vi "8HP_Clone.vi"(0 "Single 8HP":T1) -> (2 "DAQ Error":errorcluster, 3 "All samples out":sgl[][](array[numeric]), 4 "Ch No":i16[](array[numeric]), 5 "Index":i32[](array[numeric]), 6 "Sampling Rate Hz":dbl)   [LabVIEW 2018]
doc: "Use this plug-in with the Nathan 7609 data acquisition system"
uses:
  Device ID port info.ctl
  ctls/8HP_Cmd (USB).ctl
  Globals/Meas_global.vi
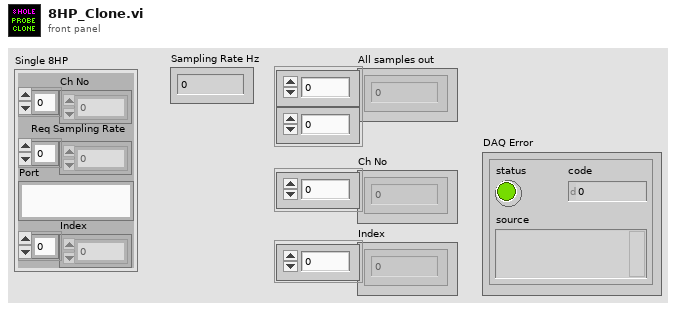
[diagram p1: front panel]
types:
  T1 = typedef "Device ID port info.ctl" = cluster{"Ch No":i16[], "Req Sampling Rate":dbl[], "Port":string, "Index":i32[]}
  T2 = typedef "8HP_Cmd (USB).ctl" = string
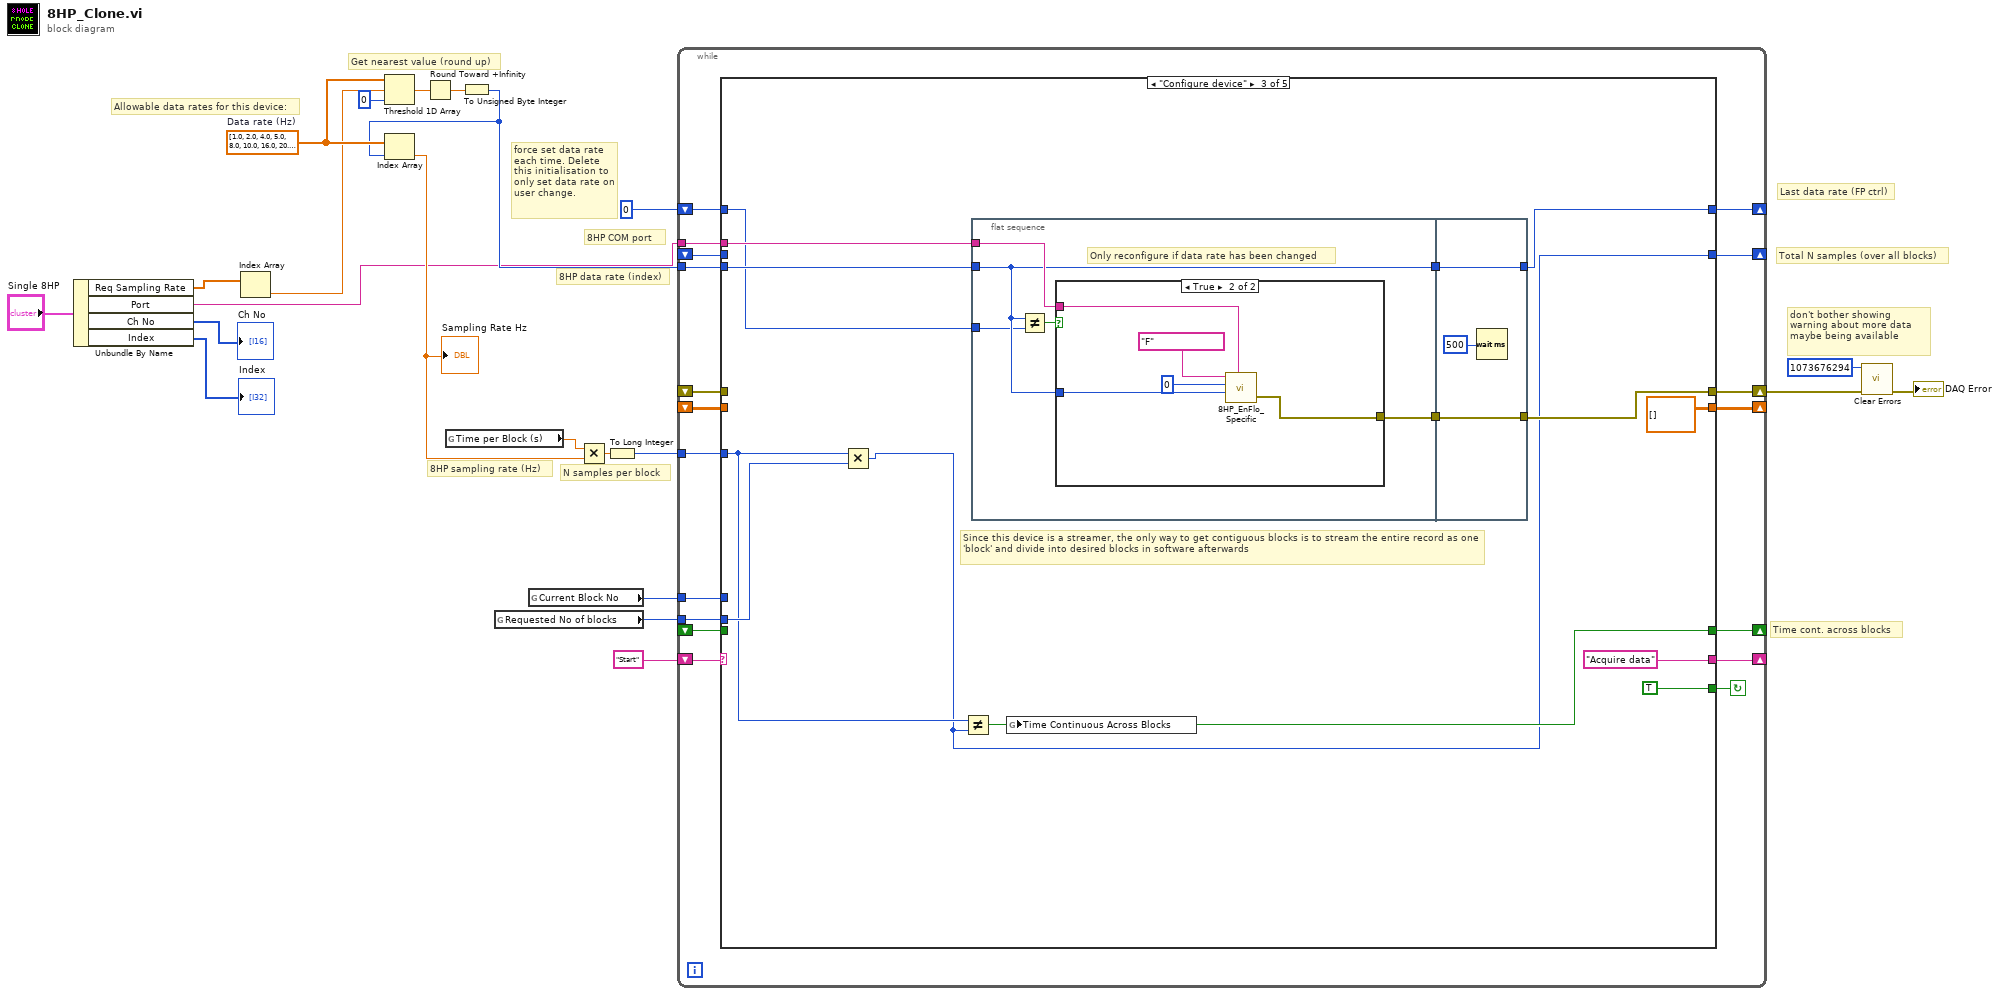
[diagram p0: block diagram]
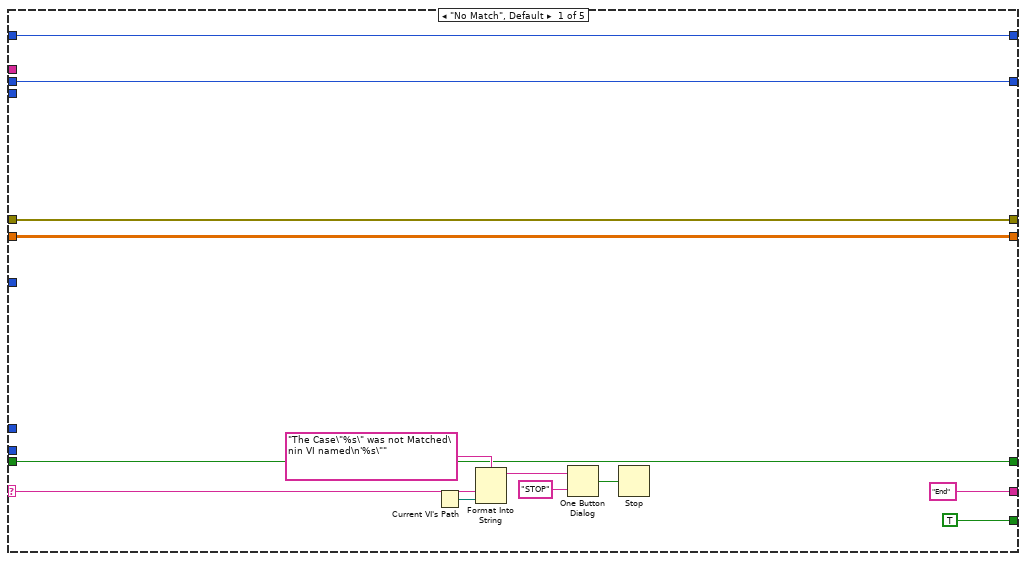
[diagram p2: hidden frame]
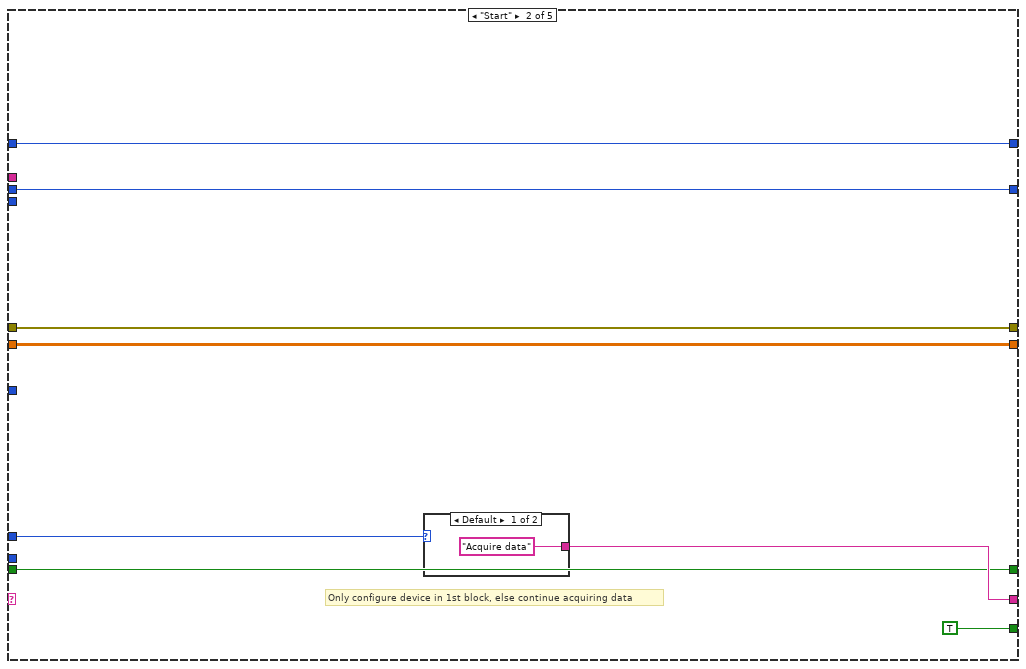
[diagram p3: hidden frame]
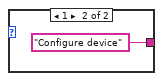
[diagram p4: hidden frame]
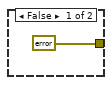
[diagram p5: hidden frame]
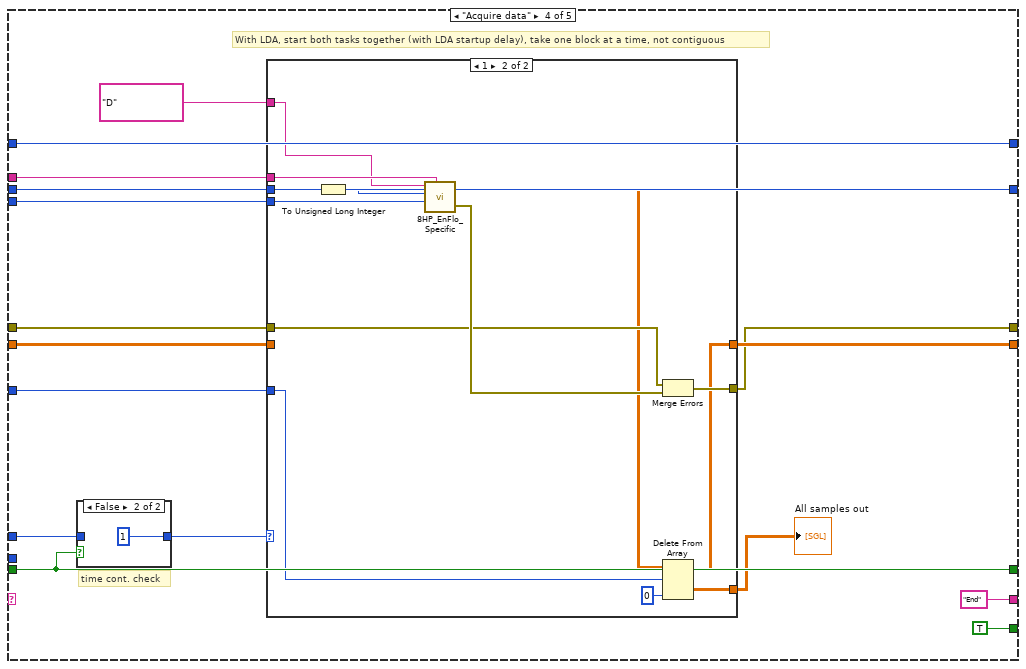
[diagram p6: hidden frame]
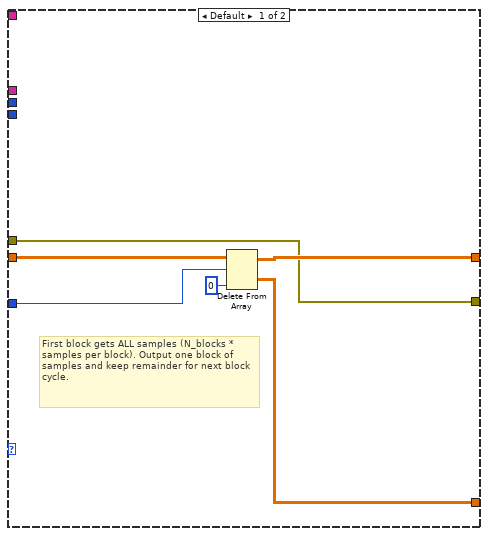
[diagram p8: hidden frame]
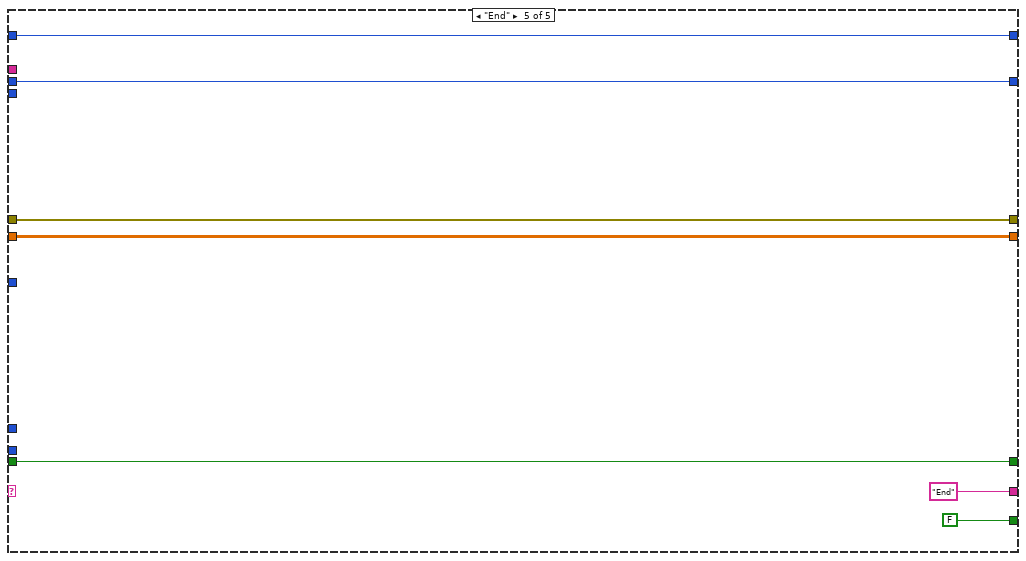
[diagram p9: hidden frame]
diagram:
  w13 = dbl[] [1.0, 2.0, 4.0, 5.0, 8.0, 10.0, 16.0, 20.0, 25.0, 32.0, 40.0, 50.0, 64.0, 80.0, 100.0, 125.0, 160.0, 200.0, 250.0, 320.0, 400.0, 500.0, 625.0, 800.0, 1000.0]  # Data rate (Hz)
  # "N samples per block"
  # "8HP sampling rate (Hz)"
  # "8HP COM port"
  # "8HP data rate (index)"
  # "Allowable data rates for this device:"
  # "Get nearest value (round up)"
  # "force set data rate each time. Delete this initialisation to only set data rate on user change."
  # "Last data rate (FP ctrl)"
  # "Total N samples (over all blocks)"
  # "don't bother showing warning about more data maybe being available"
  # "Time cont. across blocks"
  n1 = Unbundle By Name("Single 8HP") -> ("Req Sampling Rate"=w4:dbl[], "Port"=w5:string, "Ch No"=→"Ch No":i16[], "Index"=→"Index":i32[])
  n2 = Index Array(array=w4) -> (element=w3:dbl)  [unwired: 1 in]
  n3 = Threshold 1D Array(1:0 ("start index (0)"), 2:w3, 3:w13) -> (0:w14:dbl)
  n4 = Round Toward +Infinity(x=w14) -> (ceil(x): smallest int >= x=w12:dbl)
  n5 = global read "Meas_global.vi" "Time per Block (s)"() -> (w11:dbl)
  n6 = To Unsigned Byte Integer(number=w12) -> (unsigned 8bit integer=w7:u8)
  n7 = Index Array(array=w13, index=w7) -> (element=w8:dbl)
  "Sampling Rate Hz" <- w8
  n8 = global read "Meas_global.vi" "Requested No of blocks"() -> (w20:i32)
  n9 = global read "Meas_global.vi" "Current Block No"() -> (w21:i32)
  n10 = Multiply(x=w11, y=w8) -> (x*y=w10:dbl)
  n11 = To Long Integer(number=w10) -> (32bit integer=w9:i32)
  n12 = while {
    shift-left: "Start" -> [w40]
    shift-right: [w31] -> _
    tunnel: w9 -> [w39]
    tunnel: w21 -> [w38]
    tunnel: w20 -> [w36]
    shift-right: [w34] -> w17
    shift-left: _ -> [w35]
    shift-right: [w33] -> _
    shift-left: _ -> [w32]
    shift-right: [w30] -> _
    shift-left: _ -> [w29]
    tunnel: w5 -> [w28]
    tunnel: w7 -> [w27]
    shift-right: [w26] -> _
    shift-left: _ -> [w25]
    shift-right: [w24] -> _
    shift-left: u8 0 ("Pressure data rate (Hz)") -> [w23]
    stop <- w37 continue-if-true
    n13 = case shown="\"Configure device\"" w40 {
      selector: w40 -> [w46 _ _ _ _]
      tunnel: ["End" w58 "Acquire data" ("f") "End" "End" ("f")] -> w31
      tunnel: w39 -> [_ _ w72 w98 _]
      tunnel: w38 -> [_ w59 _ w101 _]
      tunnel: [TRUE TRUE TRUE TRUE FALSE] -> w37
      tunnel: w36 -> [_ _ w76 _ _]
      tunnel: w35 -> [w45 w60 _ w105 w131]
      tunnel: [w45 w60 w75 w99 w131] -> w34
      tunnel: [w44 w57 sgl[][] [] ("Channel volts") w103 w133] -> w33
      tunnel: w32 -> [w44 w57 _ w104 w133]
      tunnel: [w43 w56 w71 w100 w132] -> w30
      tunnel: w29 -> [w43 w56 _ w100 w132]
      tunnel: w28 -> [_ _ w70 w97 _]
      tunnel: w27 -> [_ _ w69 w96 _]
      tunnel: [w41 w54 w66 w94 w129] -> w26
      tunnel: w25 -> [w41 w54 _ w94 w129]
      tunnel: [w42 w55 w68 w95 w130] -> w24
      tunnel: w23 -> [w42 w55 w67 w95 w130]
      frame "No Match", Default {
        n14 = Current VI's Path() -> (path=w49:path)
        n15 = Format Into String(format string="The Case\"%s\" was not Matched\nin VI named\n'%s\"" ("Format String"), w46, w49) -> (resulting string=w52:string)  [unwired: 2 in, 1 out]
        n16 = One Button Dialog(message=w52, button name ("OK")="STOP") -> (true=w50:bool)
        n17 = Stop(stop? (T)=w50) -> ()
      }
      frame "Start" {
        # "Only configure device in 1st block, else continue acquiring data"
        n18 = case shown="Default" w59 {
          tunnel: ["Acquire data" ("f") "Configure device" ("f")] -> w58
          frame Default {
          }
          frame 1 {
          }
        }
      }
      frame "Configure device" {
        # "Since this device is a streamer, the only way to get contiguous blocks is to stream the entire record as one 'block' and divide into desired blocks in software afterwards"
        n19 = Multiply(x=w72, y=w76) -> (x*y=w66:i32)
        n20 = Not Equal?(x=w72, y=w66) -> (x != y?=w71:bool)
        n21 = flat-sequence {
          tunnel: w70 -> [w81]
          tunnel: w69 -> [w79]
          tunnel: w67 -> [w78]
          tunnel: [w82] -> w65
          tunnel: [w79] -> w64
          tunnel: [w90] -> w68
          tunnel: [w91] -> w75
          tunnel: w65 -> [w91]
          tunnel: w64 -> [w90]
          frame #0 {
            # "Only reconfigure if data rate has been changed"
            n22 = Not Equal?(x=w79, y=w78) -> (x != y?=w80:bool)
            n23 = case shown="True" w80 {
              tunnel: [errorcluster {"status"=FALSE, "code"=0, "source"=""} ("error IO") w85] -> w82
              tunnel: w81 -> [_ w84]
              tunnel: w79 -> [_ w86]
              frame False {
              }
              frame True {
                n24 = call "8HP_EnFlo_Specific.vi"("COM port"=w84, "Set data rate (Hz)"=w86, "N samples"=u32 0, "Command"=T2 "F") -> ("Error"=w85:errorcluster)  [unwired: 2 in, 1 out]
              }
            }
          }
          frame #1 {
            n25 = Wait (ms)(milliseconds to wait=u32 500) -> ()  [unwired: 1 out]
          }
        }
        n26 = global write "Meas_global.vi" "Time Continuous Across Blocks"(w71) -> ()
      }
      frame "Acquire data" {
        # "time cont. check"
        # "With LDA, start both tasks together (with LDA startup delay), take one block at a time, not contiguous"
        n27 = case shown="False" w100 {
          tunnel: [w108 1 ("Current Block No")] -> w102
          tunnel: w101 -> [w108 _]
          frame True {
          }
          frame False {
          }
        }
        n28 = case shown="1" w102 {
          tunnel: w105 -> [w111 w127]
          tunnel: [w111 w126] -> w99
          tunnel: [w113 w123] -> w103
          tunnel: w98 -> [w112 w124]
          tunnel: w104 -> [w114 _]
          tunnel: [w110 w121] -> w92
          tunnel: w97 -> [_ w120]
          tunnel: w96 -> [_ w119]
          tunnel: w94 -> [_ w118]
          tunnel: T2 "D" ("Command") -> [_ w117]
          frame Default {
            # "First block gets ALL samples (N_blocks * samples per block). Output one block of samples and keep remainder for next block cycle."
            n29 = Delete From Array(array=w114, length=w112, index (col)=0 ("disabled index (col)")) -> (deleted portion=w110:sgl[][], array with subset deleted=w113:sgl[][])  [unwired: 1 in]
          }
          frame 1 {
            n30 = To Unsigned Long Integer(number=w118) -> (unsigned 32bit integer=w116:u32)
            n31 = call "8HP_EnFlo_Specific.vi"("COM port"=w120, "Set data rate (Hz)"=w119, "N samples"=w116, "Command"=w117) -> ("Error"=w128:errorcluster, "All samples out"=w125:sgl[][])  [unwired: 2 in]
            n32 = Merge Errors(w127, w128) -> (w126:errorcluster)
            n33 = Delete From Array(array=w125, length=w124, index (col)=0 ("disabled index (col)")) -> (deleted portion=w121:sgl[][], array with subset deleted=w123:sgl[][])  [unwired: 1 in]
          }
        }
        "All samples out" <- w92
      }
      frame "End" {
      }
    }
  }
  n34 = call <vilib>:"Clear Errors.vi"("error in (no error)"=w17, "specific error code to clear (0: all)"=1073676294) -> ("error out"=→"DAQ Error":errorcluster)  [unwired: 4 in, 1 out]
